vi "case_structure_test.vi"() -> ()   [LabVIEW 2010]
panel:
  out "String 2":string
  in  "String":string
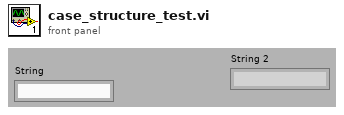
[diagram p1: front panel]
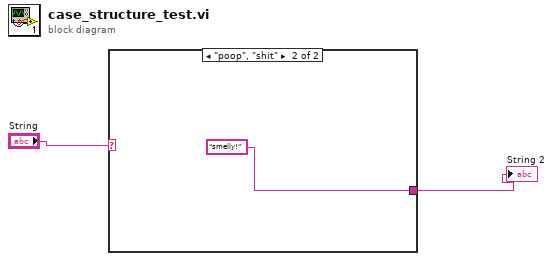
[diagram p0: block diagram]
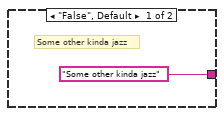
[diagram p2: hidden frame]
diagram:
  n1 = case shown="\"poop\", \"shit\"" "String" {
    tunnel: ["Some other kinda jazz" "smelly!"] -> w1
    frame "False", Default {
      # "Some other kinda jazz"
    }
    frame "poop", "shit" {
    }
  }
  "String 2" <- w1
